vi "Ejercicio 1.2.6.vi"() -> ()   [LabVIEW 2013]
panel:
  out "Boolean 2":bool
  in  "Boolean":bool
  in  "String 2":string
  out "String":string
  in  "Numeric 4":i32
  out "Numeric 3":i32
  out "Numeric 2":dbl
  in  "Numeric":dbl
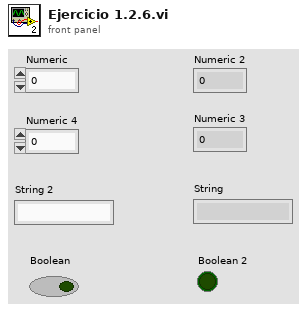
[diagram p1: front panel]
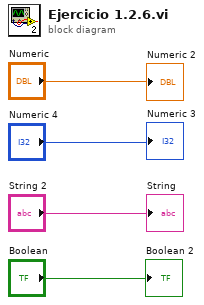
[diagram p0: block diagram]
diagram:
  "Numeric 2" <- "Numeric"
  "Numeric 3" <- "Numeric 4"
  "String" <- "String 2"
  "Boolean 2" <- "Boolean"
